vi "计算点至直线的垂足.vi"(8 "Error In":errorcluster caption="错误输入", 10 "Point":T2 caption="直线外点", 11 "直线":T1) -> (0 "Error Out":errorcluster caption="错误输出", 3 "垂足点":T2 caption="垂足")   [LabVIEW 2012, in "几何工具.lvlib"]
uses:
  <vilib>/Utility/miscctls.llb/LVPointDoubleTypeDef.ctl
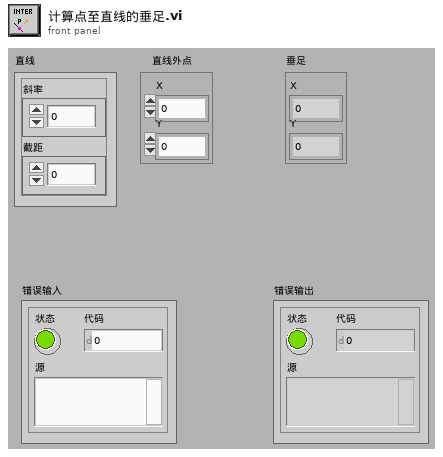
[diagram p1: front panel]
types:
  T1 = typedef "几何工具.lvlib/斜率与截距.ctl" = cluster{"斜率":dbl, "截距":dbl}
  T2 = typedef "LVPointDoubleTypeDef.ctl" = cluster{"X":dbl, "Y":dbl}
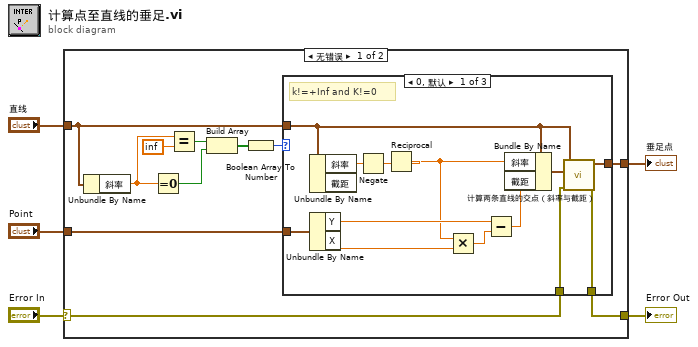
[diagram p0: block diagram]
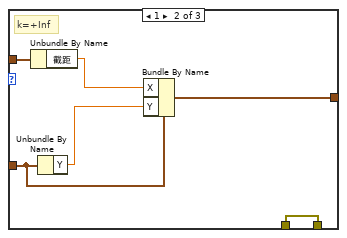
[diagram p2: hidden frame]
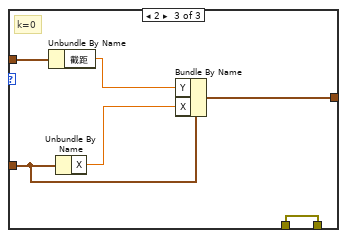
[diagram p3: hidden frame]
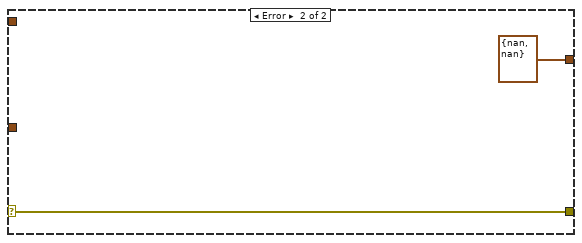
[diagram p4: hidden frame]
diagram:
  n1 = case shown="无错误" "Error In" {
    selector: "Error In" -> [w7 w43]
    tunnel: [w6 w43] -> w4
    tunnel: "直线" -> [w15 _]
    tunnel: "Point" -> [w16 _]
    tunnel: [w8 T2 {"X"=nan, "Y"=nan} ("Intersect Point")] -> w1
    frame No Error {
      n2 = Unbundle By Name(w15) -> ("斜率"=w13:dbl)
      n3 = Equal To 0?(x=w13) -> (x = 0?=w12:bool)
      n4 = Equal?(x=w13, y=inf) -> (x = y?=w11:bool)
      n5 = Build Array(w11, w12) -> (w10:bool[])
      n6 = Boolean Array To Number(Boolean array=w10) -> (number=w9:u32)
      n7 = case shown="0, 默认" w9 {
        tunnel: [w19 w32 w39] -> w8
        tunnel: w15 -> [w22 w35 w41]
        tunnel: w16 -> [w29 w30 w40]
        tunnel: w7 -> [w18 w31 w38]
        tunnel: [w17 w31 w38] -> w6
        frame 0, Default {
          # "k!=+Inf and K!=0"
          n8 = Unbundle By Name(w22) -> ("斜率"=w28:dbl)  [unwired: 1 out]
          n9 = Unbundle By Name(w29) -> ("Y"=w24:dbl, "X"=w26:dbl)
          n10 = Negate(x=w28) -> (-x=w27:dbl)
          n11 = Reciprocal(x=w27) -> (1/x=w23:dbl)
          n12 = Multiply(x=w23, y=w26) -> (x*y=w25:dbl)
          n13 = Subtract(x=w24, y=w25) -> (x-y=w21:dbl)
          n14 = Bundle By Name(cluster=w22, "斜率"=w23, "截距"=w21) -> (w20:T1)
          n15 = call "计算两条直线的交点（斜率与截距）.vi"("Error In"=w18, "直线B"=w20, "直线A"=w22) -> ("Error Out"=w17:errorcluster, "交点"=w19:T2)  [unwired: 7 in]
        }
        frame 1 {
          # "k=+Inf"
          n16 = Unbundle By Name(w35) -> ("截距"=w34:dbl)
          n17 = Unbundle By Name(w30) -> ("Y"=w33:dbl)
          n18 = Bundle By Name(cluster=w30, "X"=w34, "Y"=w33) -> (w32:T2)
        }
        frame 2 {
          # "k=0"
          n19 = Unbundle By Name(w41) -> ("截距"=w37:dbl)
          n20 = Unbundle By Name(w40) -> ("X"=w36:dbl)
          n21 = Bundle By Name(cluster=w40, "Y"=w37, "X"=w36) -> (w39:T2)
        }
      }
    }
    frame Error {
    }
  }
  "Error Out" <- w4
  "垂足点" <- w1
